vi "Triton_temp_code.vi"() -> (0 "String":string)   [LabVIEW 2021]
panel:
  in  "Temperature Channel":i32=8
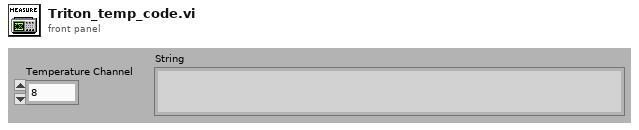
[diagram p1: front panel]
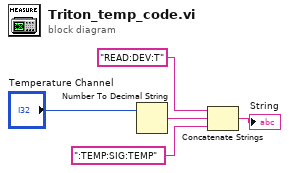
[diagram p0: block diagram]
diagram:
  n1 = Number To Decimal String(number="Temperature Channel") -> (decimal integer string=w1:string)  [unwired: 1 in]
  n2 = Concatenate Strings("READ:DEV:T", w1, ":TEMP:SIG:TEMP") -> (→"String":string)
